vi "NI VeriStand - Run Macro Player.vi"(8 "error in (no error)":errorcluster, 10 "Play Mode":T1, 11 "MacroPlayer in":T2) -> (0 "error out":errorcluster, 3 "MacroPlayer out":T2)   [LabVIEW 2020, in "NI_VS MacroPlayerAPI.lvlib"]
doc: "Runs the Macro Player tool and specifies the speed at which to play back macro files you record using the Macro Recorder VIs or the Macro Recorder tool in NI VeriStand."
uses:
  <vilib>/NI VeriStand/Execution/MacroPlayer/NI_VS MacroPlayerAPI.lvlib
  <vilib>/NI VeriStand/Execution/MacroPlayer/MacroPlayerAPI.ctl
  NationalInstruments.VeriStand.ClientAPI
  <vilib>/NI VeriStand/Execution/MacroPlayer/Play Mode.ctl
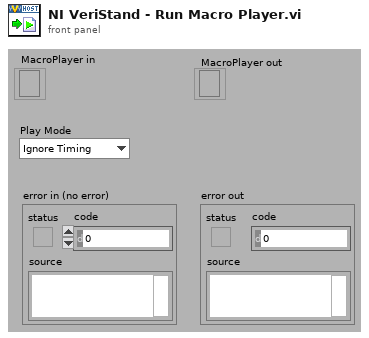
[diagram p1: front panel]
types:
  T1 = typedef "NI_VS MacroPlayerAPI.lvlib/Play Mode.ctl" = enum8{"Ignore Timing", "Use Timing"}
  T2 = typedef "NI_VS MacroPlayerAPI.lvlib/MacroPlayerAPI.ctl" = refnum<k24>
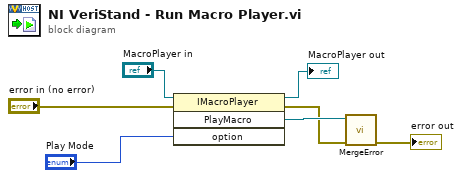
[diagram p0: block diagram]
diagram:
  n1 = invoke class="IMacroPlayer" method="PlayMacro"(reference="MacroPlayer in", error in="error in (no error)", "option"="Play Mode") -> (reference out=→"MacroPlayer out":T2, error out=w2:errorcluster, "PlayMacro"=w3:refnum<k24>)  [unwired: 1 in, 1 out]
  n2 = call <vilib>:"MergeError.vi"("error in (no error)"=w2, "Error"=w3) -> ("error out"=→"error out":errorcluster)  [unwired: 9 out]
